vi "Arduino_SetBAUD.vi"(8 "error in (no error)":errorcluster, 11 "Arduino In":T1={"Java"=path "/Applications/Arduino.app/Contents/Java", "Packages"=path "/Users/crogers/Library/Arduino15/packages", "folder"=path "/Users/crogers/Documents/LabVIEW Data", "serial"="/dev/cu.usbmodem14301", "Console"=""}) -> (0 "error out":errorcluster, 3 "Arduino Out":T1={"Java"=path "/Applications/Arduino.app/Contents/Java", "Packages"=path "/Users/crogers/Library/Arduino15/packages", "folder"=path "/Users/crogers/Documents/LabVIEW Data", "serial"="/dev/cu.usbmodem14301", "Console"=""})   [LabVIEW 2020]
uses:
  Arduino.ctl
panel:
  out "error out":errorcluster
  in  "error in (no error)":errorcluster
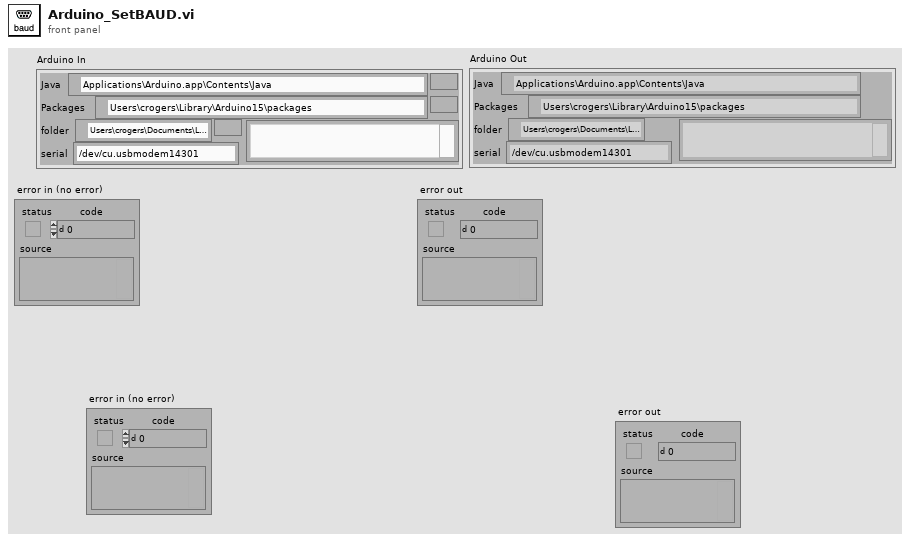
[diagram p1: front panel]
types:
  T1 = typedef "Arduino.ctl" = cluster{"Java":path, "Packages":path, "folder":path, "serial":string, "Console":string}
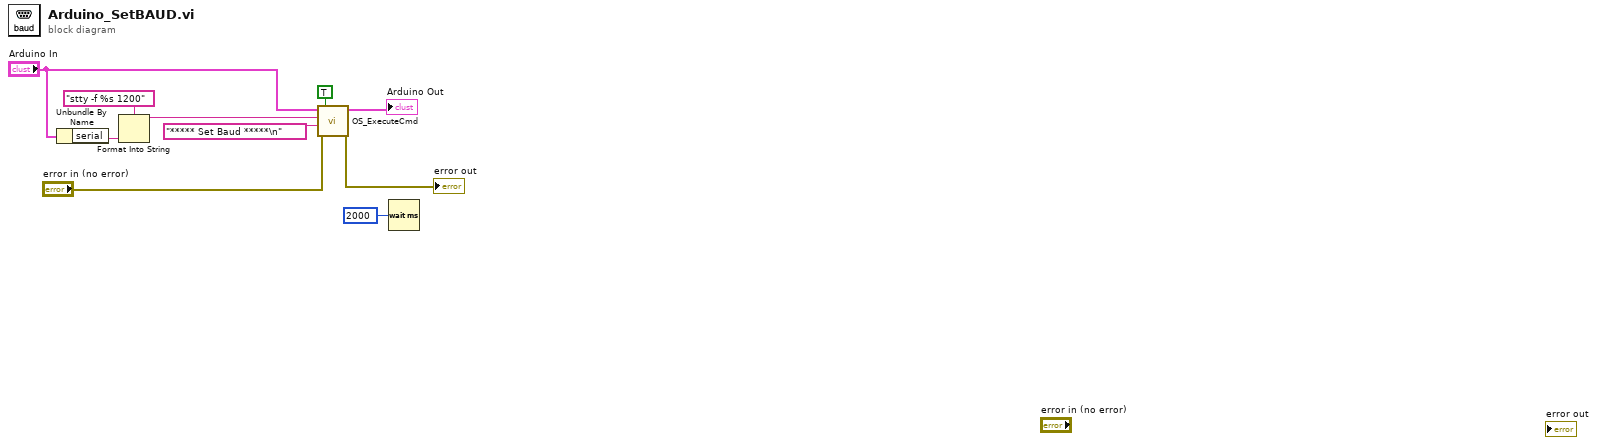
[diagram p0: block diagram]
diagram:
  n1 = Unbundle By Name("Arduino In") -> ("serial"=w10:string)
  n2 = Format Into String(format string="stty -f %s 1200" ("string"), w10) -> (resulting string=w3:string)  [unwired: 2 in, 1 out]
  n3 = call "OS_ExecuteCmd.vi"("wait until completion? (T)"=TRUE, "error in (no error)"="error in (no error)", "Comment"="***** Set Baud *****\n" ("string"), "Command"=w3, "Arduino In"="Arduino In") -> ("error out"=→"error out":errorcluster, "Arduino out"=→"Arduino Out":T1)  [unwired: 5 in]
  n4 = Wait (ms)(milliseconds to wait=u32 2000) -> ()  [unwired: 1 out]
